vi "write to fifo.vi"(0 "5785_3.2GHz_one channel in":refnum<class "5785_3.2GHz_one channel.lvclass">, 11 "error in (no error)":errorcluster) -> (4 "5785_3.2GHz_one channel out":refnum<class "5785_3.2GHz_one channel.lvclass">, 6 "done write file":bool=TRUE, 8 "num of pulses sent to the FPGA":u32, 10 "room on fifo":bool=TRUE, 15 "error out":errorcluster)   [LabVIEW 2021, in "5785_3.2GHz_one channel.lvclass"]
uses:
  5785_3.2GHz_one channel.lvclass
  5785_3.2GHz_one channel.lvclass/5785_3.2GHz_one channel.ctl
  <vilib>/Utility/error.llb/Error Cluster From Error Code.vi
  <vilib>/rvi/errors/niLvFpgaAdjustHostInterfaceError.vi
  <vilib>/rvi/interface/nirviMethod/nirviMethod.xnode
  <vilib>/FPGAPlugInAG/Dynamic/niLvFpga_WriteFifo_Dynamic.vi
  <vilib>/rvi/errors/niLvFpgaMergeErrorWithErrorCode.vi
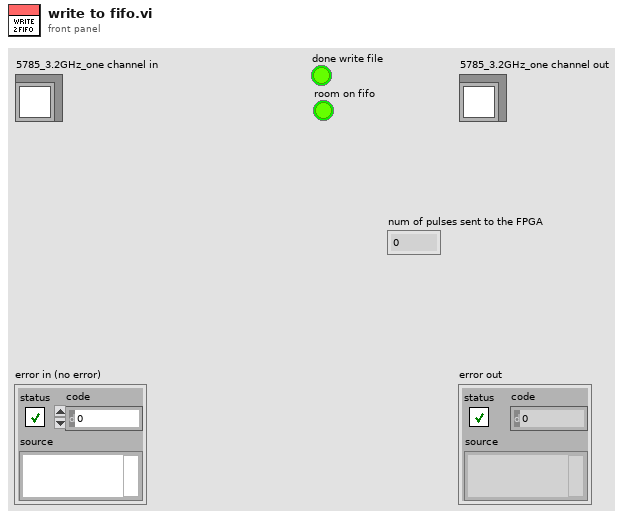
[diagram p1: front panel]
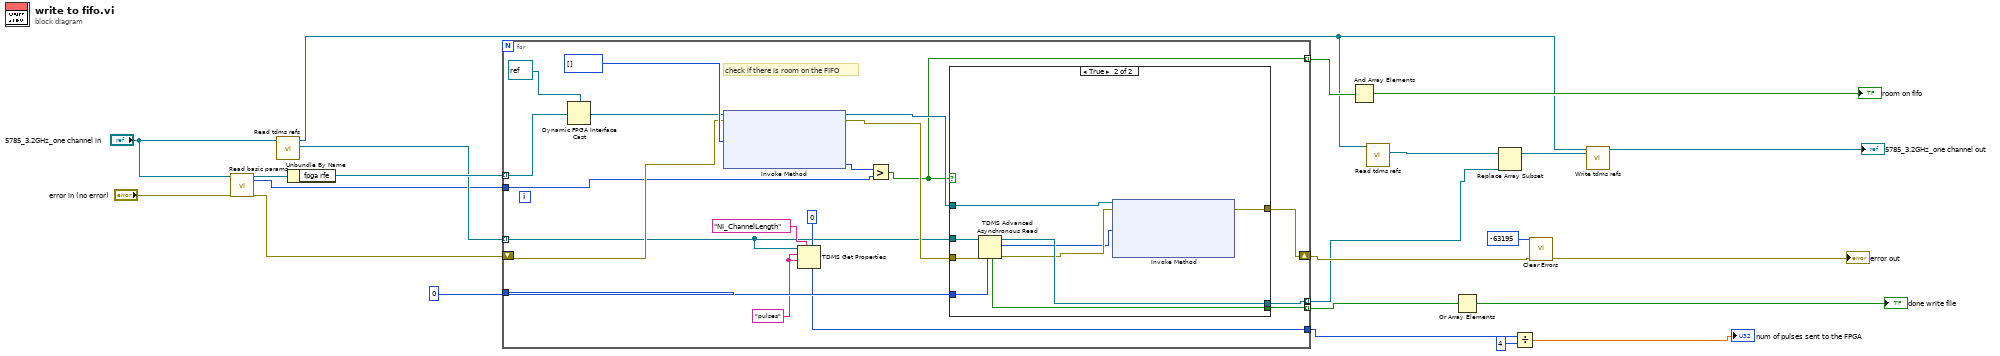
[diagram p0: block diagram]
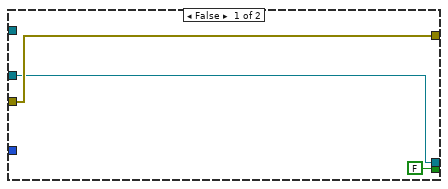
[diagram p2: hidden frame]
diagram:
  n1 = call-dynamic "Read basic params.vi"("device_type in"="5785_3.2GHz_one channel in", "error in (no error)"="error in (no error)") -> ("device_type out"=w10:refnum<class "5785_3.2GHz_one channel.lvclass">, "buffer size"=w12:u32, "error out"=w8:errorcluster)  [unwired: 12 in, 3 out]
  n2 = call-dynamic "Read tdms refs.vi"("device_type in"="5785_3.2GHz_one channel in") -> ("tdms refs"=w13:refnum<k34>[], "device_type out"=w6:refnum<class "5785_3.2GHz_one channel.lvclass">)  [unwired: 8 in, 1 out]
  n3 = Unbundle By Name(w10) -> ("fpga rfe"=w21:refnum<k20>[])
  n4 = for {
    tunnel: w13 -> [w25] mode=indexing
    tunnel: w21 -> [w31] mode=indexing
    tunnel: u64 0 ("type") -> [w42]
    tunnel: [w41] -> w22 mode=indexing
    tunnel: [w40] -> w17 mode=indexing
    shift-right: [w39] -> w19
    shift-left: w8 -> [w37]
    tunnel: w12 -> [w36]
    tunnel: [w33] -> w18 mode=indexing
    tunnel: [w24] -> w3
    w26 = "pulses" ("channel name")
    # "check if there is room on the FIFO"
    n5 = Dynamic FPGA Interface Cast(Session In=refnum<k20> refnum ("FPGA VI Reference Out"), Type=w31) -> (Session Out=w30:refnum<k20>)
    n6 = xnode "Invoke Method"("FPGA VI Reference In"=w30, "error in"=w37, "Data"=u64[] []) -> ("FPGA VI Reference Out"=w34:refnum<k20>, "error out"=w35:errorcluster, "Empty Elements Remaining"=w32:u32)  [unwired: 1 in]
    n7 = TDMS Get Properties(5:u64 0, 7:"NI_ChannelLength" ("property name"), 9:w26, 10:w26, 11:w25) -> (4:w24:u64)  [unwired: 1 in, 5 out]
    n8 = Greater?(x=w32, y=w36) -> (0:w33:bool)
    n9 = case shown="True" w33 {
      tunnel: w25 -> [w44 w54]
      tunnel: w42 -> [_ w53]
      tunnel: [FALSE ("read process finished?") w52] -> w41
      tunnel: [w44 w51] -> w40
      tunnel: [w45 w49] -> w39
      tunnel: w35 -> [w45 w48]
      tunnel: w34 -> [_ w47]
      frame False {
      }
      frame True {
        n10 = TDMS Advanced Asynchronous Read(6:w53, 8:w48, 11:w54) -> (0:w50:errorcluster, 2:w46:u64[], 3:w51:refnum<k34>, 4:w52:bool)
        n11 = xnode "Invoke Method"("FPGA VI Reference In"=w47, "error in"=w50, "Data"=w46) -> ("error out"=w49:errorcluster)  [unwired: 1 in, 2 out]
      }
    }
  }
  n12 = And Array Elements(Boolean array=w18) -> (logical AND=→"room on fifo":bool)
  n13 = call-dynamic "Read tdms refs.vi"("device_type in"=w6) -> ("tdms refs"=w7:refnum<k34>[])  [unwired: 8 in, 2 out]
  n14 = Or Array Elements(Boolean array=w22) -> (logical OR=→"done write file":bool)
  n15 = Replace Array Subset(array=w7, new element=w17) -> (w4:refnum<k34>[])  [unwired: 1 in]
  n16 = Divide(x=w3, y=u64 4) -> (x/y=→"num of pulses sent to the FPGA":dbl)
  n17 = call <vilib>:"Clear Errors.vi"("error in (no error)"=w19, "specific error code to clear (0: all)"=-63195) -> ("error out"=→"error out":errorcluster)  [unwired: 4 in, 1 out]
  n18 = call-dynamic "Write tdms refs.vi"("tdms refs"=w4, "device_type in"=w6) -> ("device_type out"=→"5785_3.2GHz_one channel out":refnum<class "5785_3.2GHz_one channel.lvclass">)  [unwired: 8 in, 1 out]
